vi "OAT State Machine Generate Event for String.vi"(1 "Initialize":bool, 2 "String":string, 4 "Action":enum16{"Changed"}(ring)) -> (7 "Event":bool)   [LabVIEW 2017]
doc: "Detects events for the String objects. When the string is changed, the output is set as TRUE."
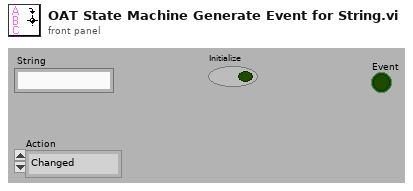
[diagram p1: front panel]
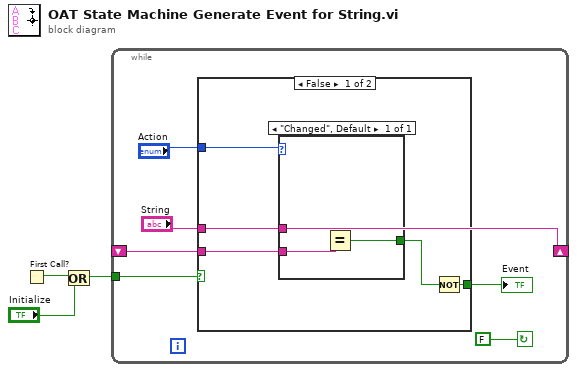
[diagram p0: block diagram]
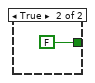
[diagram p2: hidden frame]
diagram:
  n1 = First Call?() -> (First Call?: T/F=w3:bool)
  n2 = Or(x=w3, y="Initialize") -> (x .or. y?=w1:bool)
  n3 = while {
    tunnel: w1 -> [w6]
    shift-left: _ -> [w9]
    shift-right: ["String"] -> _
    stop <- FALSE continue-if-true
    n4 = case shown="False" w6 {
      tunnel: "Action" -> [w14 _]
      tunnel: w9 -> [w13 _]
      tunnel: "String" -> [w12 _]
      tunnel: [w10 FALSE] -> w4
      frame False {
        n5 = case shown="\"Changed\", Default" w14 {
          tunnel: w12 -> [w17]
          tunnel: w13 -> [w16]
          tunnel: [w15] -> w11
          frame "Changed", Default {
            n6 = Equal?(x=w17, y=w16) -> (x = y?=w15:bool)
          }
        }
        n7 = Not(x=w11) -> (.not. x?=w10:bool)
      }
      frame True {
      }
    }
    "Event" <- w4
  }
